vi "抽奖.vi"() -> ()   [LabVIEW 2018]
panel:
  in  "布尔":bool
  out "数值":i16
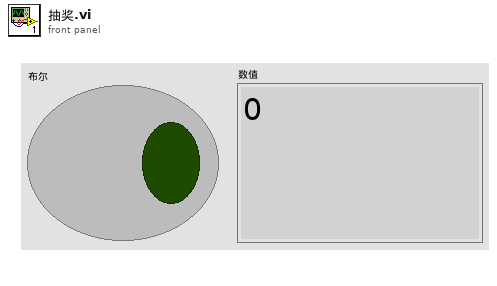
[diagram p1: front panel]
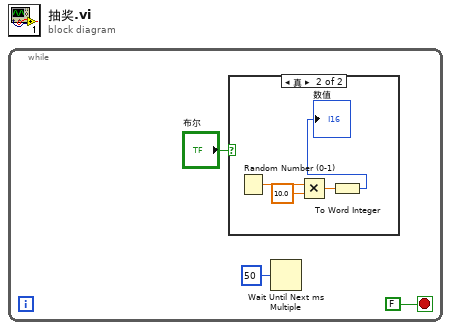
[diagram p0: block diagram]
diagram:
  n1 = while {
    stop <- FALSE stop-if-true
    n2 = case shown="真" "布尔" {
      frame False {
      }
      frame True {
        n3 = Random Number (0-1)() -> (number: 0 to 1=w7:dbl)
        n4 = Multiply(x=w7, y=10.0) -> (x*y=w5:dbl)
        n5 = To Word Integer(number=w5) -> (16bit integer=→"数值":i16)
      }
    }
    n6 = Wait Until Next ms Multiple(millisecond multiple=u32 50 ("毫秒倍数")) -> ()  [unwired: 1 out]
  }
